vi "check_path.vi"(4 "error in":errorcluster, 6 "Base_path":path, 7 "Config_Path":path=path "../configurations/open_sense/sensors_config.json") -> (0 "error out":errorcluster, 3 "Config_path_out":path=path "../configurations/open_sense/sensors_config.json")   [LabVIEW 2019]
doc: "Check if a path is relative or absolute. Decide to pass the name of the file or the path."
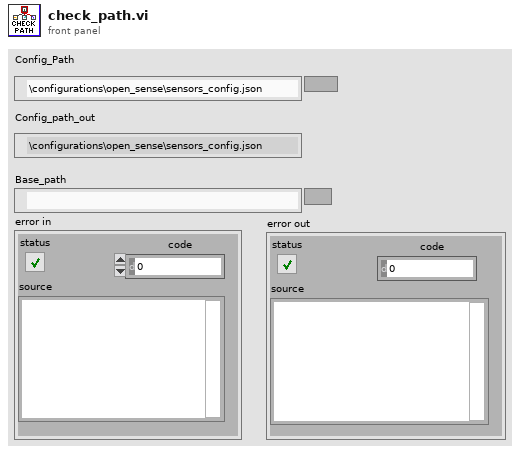
[diagram p1: front panel]
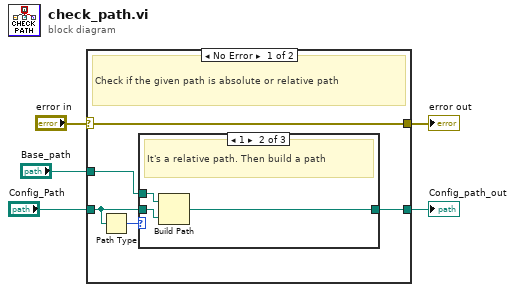
[diagram p0: block diagram]
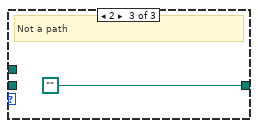
[diagram p3: hidden frame]
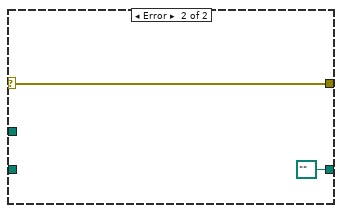
[diagram p4: hidden frame]
diagram:
  n1 = case shown="No Error" "error in" {
    selector: "error in" -> [w9 w17]
    tunnel: [w9 w17] -> w4
    tunnel: "Base_path" -> [w7 _]
    tunnel: [w8 path "" ("appended path")] -> w3
    tunnel: "Config_Path" -> [w6 _]
    frame No Error {
      # "Check if the given path is absolute or relative path"
      n2 = Path Type(1:w6) -> (0:w10:i16)
      n3 = case shown="1" w10 {
        tunnel: [w11 w13 path ""] -> w8
        tunnel: w6 -> [w11 w12 _]
        tunnel: w7 -> [_ w14 _]
        frame 0, Default {
          # "It is an absolute path"
        }
        frame 1 {
          # "It's a relative path. Then build a path"
          n4 = Build Path(base path=w14, name or relative path=w12) -> (appended path=w13:path)
        }
        frame 2 {
          # "Not a path"
        }
      }
    }
    frame Error {
    }
  }
  "error out" <- w4
  "Config_path_out" <- w3
